vi "ma_Two-sided Power Spectrum (CDB).vi"(8 "error in":errorcluster, 10 "dt":dbl format="%0.2f", 11 "signal (V)":cdb[](array[numeric]) format="%0.2f") -> (0 "error out":errorcluster, 1 "f0":dbl format="%0.2f", 2 "df":dbl format="%0.2f", 3 "power spectrum (V^2 rms)":dbl[](array[numeric]) format="%0.2f")   [LabVIEW 2020, in "NI_MAPro.lvlib"]
uses:
  NI_MAPro.lvlib
  NI_AALPro.lvlib
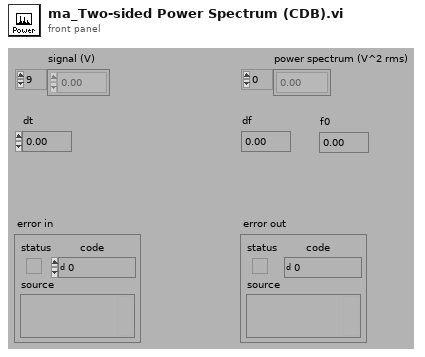
[diagram p1: front panel]
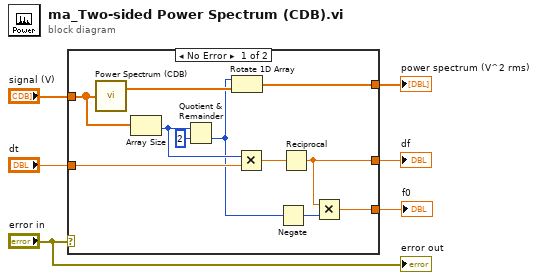
[diagram p0: block diagram]
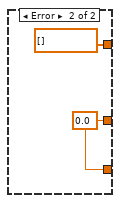
[diagram p2: hidden frame]
diagram:
  n1 = case shown="No Error" "error in" {
    tunnel: "dt" -> [w16 _]
    tunnel: "signal (V)" -> [w14 _]
    tunnel: [w9 w18] -> w4
    tunnel: [w11 dbl[] [] ("one-sided spectrum (real)")] -> w3
    tunnel: [w7 w18] -> w1
    frame No Error {
      n2 = call "Power Spectrum (CDB).vi"("X"=w14) -> ("Power Spectrum"=w13:dbl[])  [unwired: 1 out]
      n3 = Array Size(array=w14) -> (size(s)=w12:i32)
      n4 = Quotient & Remainder(x=w12, y=2) -> (floor(x/y)=w8:i32)  [unwired: 1 out]
      n5 = Rotate 1D Array(1:w13, 2:w8) -> (0:w11:dbl[])
      n6 = Multiply(x=w12, y=w16) -> (x*y=w17:dbl)
      n7 = Negate(x=w8) -> (-x=w10:i32)
      n8 = Reciprocal(x=w17) -> (1/x=w9:dbl)
      n9 = Multiply(x=w9, y=w10) -> (x*y=w7:dbl)
    }
    frame Error {
      w18 = 0.0
    }
  }
  "power spectrum (V^2 rms)" <- w3
  "df" <- w4
  "f0" <- w1
  "error out" <- "error in"
